vi "Arm.vi"(11 "input cluster":T1) -> ()   [LabVIEW 2015]
uses:
  Joystick/ControlsToCommands.ctl
  References/Refnums.vi
  Robot Global Data.vi
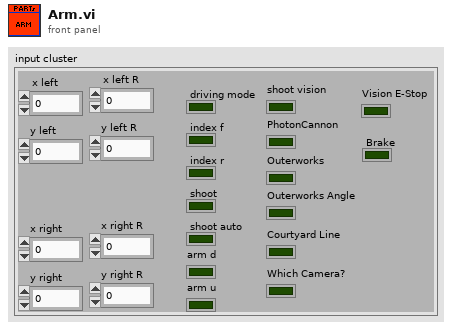
[diagram p1: front panel]
types:
  T1 = typedef "ControlsToCommands.ctl" = cluster{"x left":dbl, "y left":dbl, "x right":dbl, "y right":dbl, "driving mode":bool, "index f":bool, "index r":bool, "shoot":bool, "shoot auto":bool, "arm d":bool, "arm u":bool, "shoot vision":bool, "PhotonCannon":bool, "Outerworks":bool, "Outerworks Angle":bool, "Courtyard Line":bool, "Which Camera?":bool, "Vision E-Stop":bool, "x left R":dbl, "y left R":dbl, "x right R":dbl, "y right R":dbl, "Brake":bool}
  T2 = typedef "WPI_MotorControlDeviceRef.ctl" = cluster{"DeviceStatus":errorcluster, "Type":T3, "PWM":cluster{"PWM Channel":T4, "DeadBand":T5}, "CAN":cluster{"Device Number":u8, "Control Mode":T6, "Semaphore":T7, "Max Vout":dbl, "TalonSRX Control Mode":T8}, "Invert":bool}
  T3 = typedef "WPI_MotorControlType.ctl" = enum16{"PWM", "CAN", "CANTalonSRX"}
  T4 = typedef "FPGA_DIOPWMChannel.ctl" = enum8{"PWM 0", "PWM 1", "PWM 2", "PWM 3", "PWM 4", "PWM 5", "PWM 6", "PWM 7", "PWM 8", "PWM 9", "PWM MXP 0", "PWM MXP 1", "PWM MXP 2", "PWM MXP 3", "PWM MXP 4", "PWM MXP 5", "PWM MXP 6", "PWM MXP 7", "PWM MXP 8", "PWM MXP 9", "Invalid"}
  T5 = typedef "WPI_PWMDeadband.ctl" = cluster{"Name":string, "maxPositivePwm":i32, "minPositivePwm":i32, "centerPwm":i32, "maxNegativePwm":i32, "minNegativePwm":i32, "angularRange":u16}
  T6 = typedef "WPI_CANJaguar_ControlMode.ctl" = enum8{"Percent VBus", "Current", "Speed", "Position", "Voltage"}
  T7 = typedef "Semaphore RefNum" = refnum<k1>
  T8 = typedef "WPI_CANTalonSRX_APIControlMode.ctl" = enum8{"Percent VBus", "Speed", "Position", "Slave", "Unchanged / Invalid", "Voltage Compensation", "Current", "Motion Profile"}
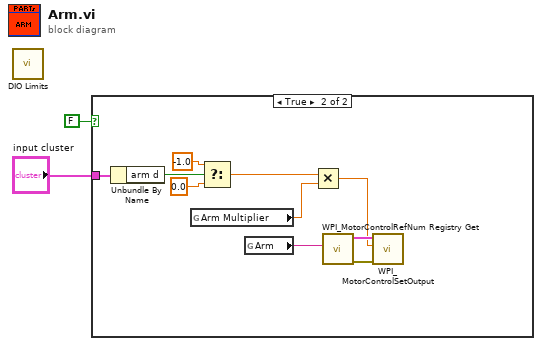
[diagram p0: block diagram]
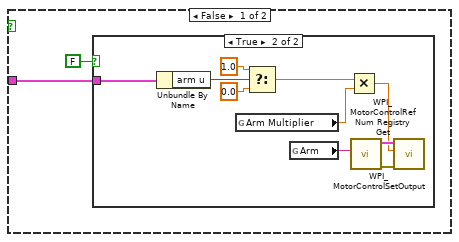
[diagram p2: hidden frame]
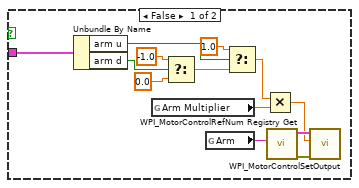
[diagram p3: hidden frame]
diagram:
  n1 = call "DIO Limits.vi"() -> ()  [unwired: 10 in, 2 out]
  n2 = case shown="True" FALSE {
    tunnel: "input cluster" -> [w4 w31]
    frame False {
      n3 = case shown="True" FALSE {
        tunnel: w4 -> [w10 w23]
        frame False {
          n4 = Unbundle By Name(w10) -> ("arm u"=w5:bool, "arm d"=w6:bool)
          n5 = global read "Robot Global Data.vi" "Arm Multiplier"() -> (w9:dbl)
          n6 = Select(t=-1.0, s=w6, f=0.0) -> (s? t:f=w12:dbl)
          n7 = global read "Refnums.vi" "Arm"() -> (w17:string)
          n8 = Select(t=1.0, s=w5, f=w12) -> (s? t:f=w8:dbl)
          n9 = Multiply(x=w8, y=w9) -> (x*y=w7:dbl)
          n10 = call <vilib>:"WPI_MotorControlRefNum Registry Get.vi"("refnum name"=w17) -> ("error out"=w11:errorcluster, "MotorControlDevRef"=w16:T2)  [unwired: 9 in]
          n11 = call <vilib>:"WPI_MotorControlSetOutput.vi"("error in (no error)"=w11, "Output"=w7, "MotorControlDevRef"=w16) -> ()  [unwired: 6 in, 3 out]
        }
        frame True {
          n12 = Unbundle By Name(w23) -> ("arm u"=w21:bool)
          n13 = global read "Robot Global Data.vi" "Arm Multiplier"() -> (w20:dbl)
          n14 = Select(t=1.0, s=w21, f=0.0) -> (s? t:f=w19:dbl)
          n15 = global read "Refnums.vi" "Arm"() -> (w27:string)
          n16 = Multiply(x=w19, y=w20) -> (x*y=w18:dbl)
          n17 = call <vilib>:"WPI_MotorControlRefNum Registry Get.vi"("refnum name"=w27) -> ("error out"=w24:errorcluster, "MotorControlDevRef"=w26:T2)  [unwired: 9 in]
          n18 = call <vilib>:"WPI_MotorControlSetOutput.vi"("error in (no error)"=w24, "Output"=w18, "MotorControlDevRef"=w26) -> ()  [unwired: 6 in, 3 out]
        }
      }
    }
    frame True {
      n19 = Unbundle By Name(w31) -> ("arm d"=w35:bool)
      n20 = global read "Robot Global Data.vi" "Arm Multiplier"() -> (w30:dbl)
      n21 = Select(t=-1.0, s=w35, f=0.0) -> (s? t:f=w29:dbl)
      n22 = global read "Refnums.vi" "Arm"() -> (w37:string)
      n23 = Multiply(x=w29, y=w30) -> (x*y=w28:dbl)
      n24 = call <vilib>:"WPI_MotorControlRefNum Registry Get.vi"("refnum name"=w37) -> ("error out"=w32:errorcluster, "MotorControlDevRef"=w36:T2)  [unwired: 9 in]
      n25 = call <vilib>:"WPI_MotorControlSetOutput.vi"("error in (no error)"=w32, "Output"=w28, "MotorControlDevRef"=w36) -> ()  [unwired: 6 in, 3 out]
    }
  }
